vi "Dual_DM_Control_Main_V3.vi"() -> ()   [LabVIEW 2014]
uses:
  Controls/MirrorModes.ctl
  Controls/Standard Action.ctl
  <vilib>/Analysis/baseanly.llb/Mean (DBL).vi
  <vilib>/Utility/file.llb/Write To Spreadsheet File (DBL).vi
  <vilib>/Utility/file.llb/Read From Spreadsheet File (DBL).vi
  <vilib>/Analysis/NI_AALBase.lvlib
panel:
  in  "Active Mirror":enum32{"Mirror 1", "Mirror 2"}(radio)
  in  "Clear Modes":bool
  in  "Mirror Modes":T1
  in  "Load Modes":bool
  in  "Save Modes":bool
  in  "Scan Modes":bool
  in  "Load Flat":bool
  in  "Apply Zero":bool
  in  "Load V Map":bool
  in  "Save V Map":bool
  in  "Apply Flat":bool
  in  "Center Bias":bool
  in  "Exit":bool
  out "Pixel Map (-1 to 1)":dbl[][](graph)
  # "Mode"
  # "Amount (nm)"
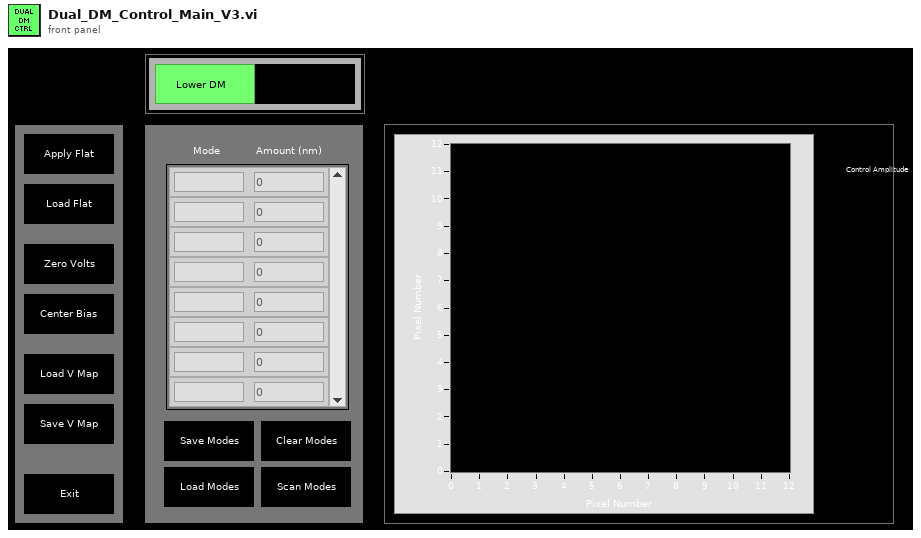
[diagram p1: front panel]
types:
  T1 = typedef "MirrorModes.ctl" = cluster{"Mode":string, "Amplitude":dbl}[]
  T2 = typedef "Standard Action.ctl" = enum16{"Read", "Write"}
  T3 = typedef "MirrorModes_DUAL.ctl" = cluster{"Mode":string, "Amplitude":dbl}[][]
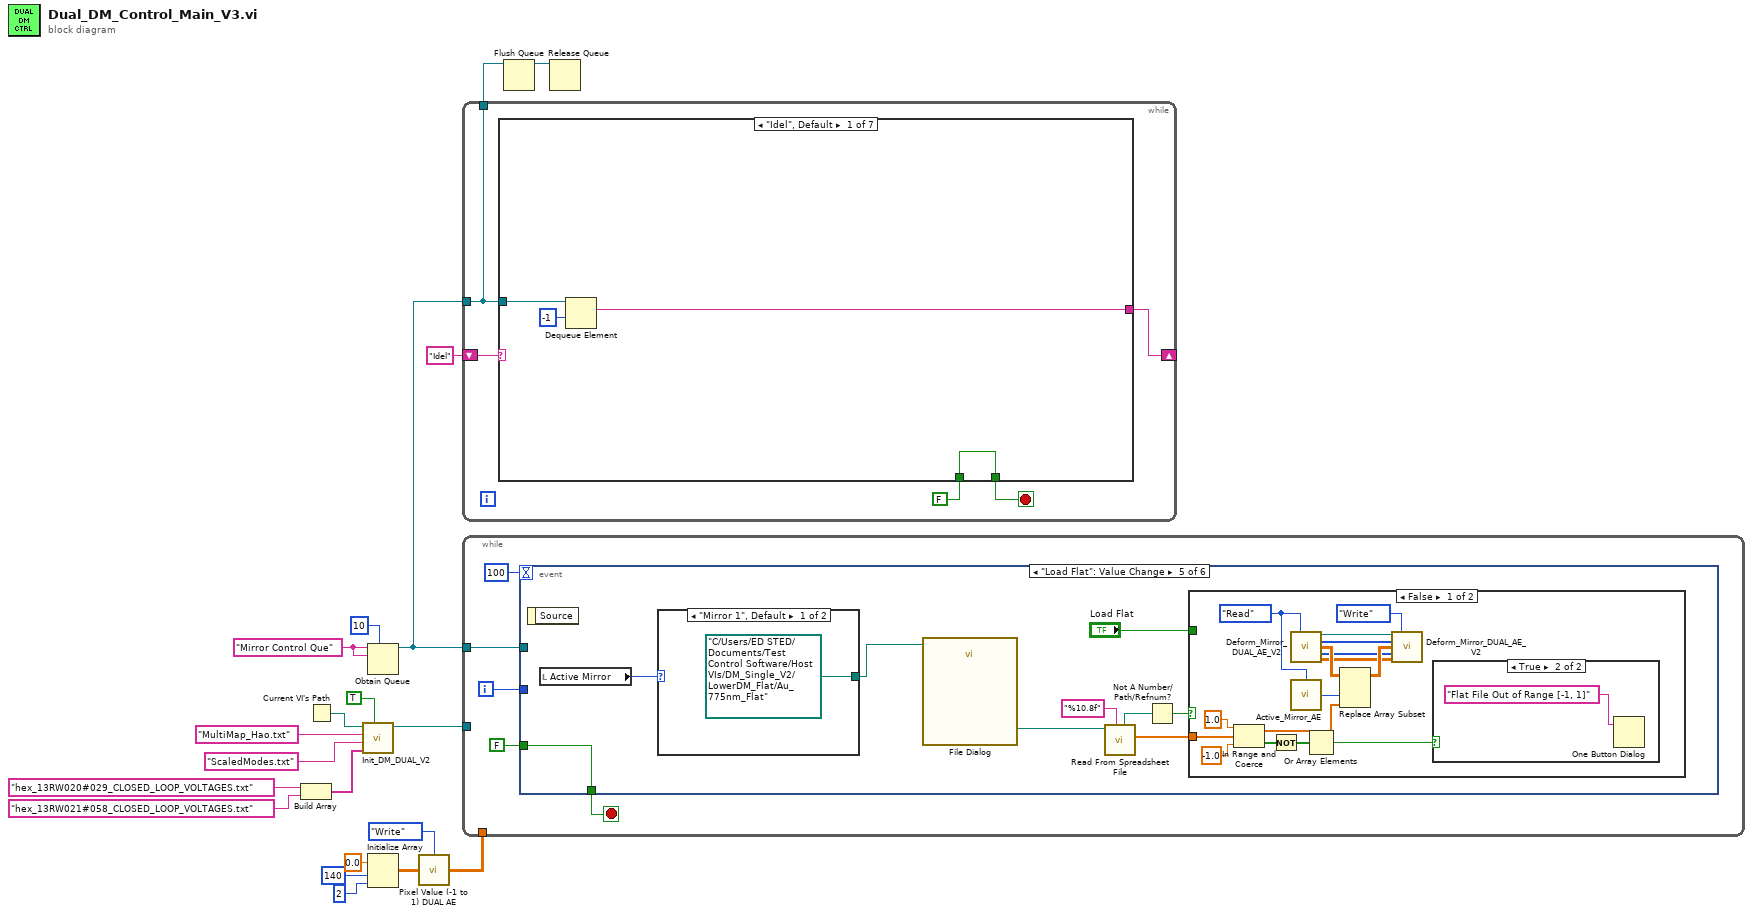
[diagram p0: block diagram]
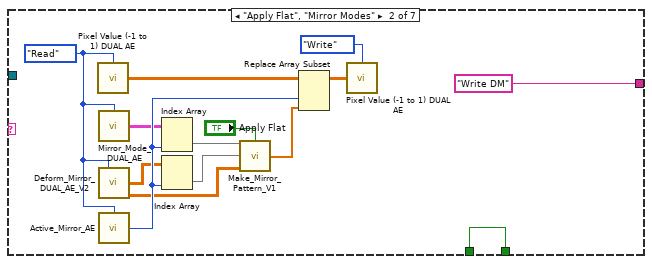
[diagram p2: hidden frame]
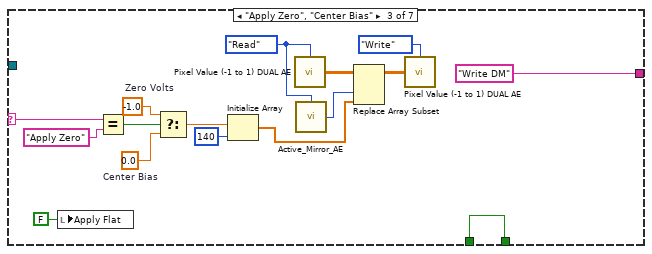
[diagram p3: hidden frame]
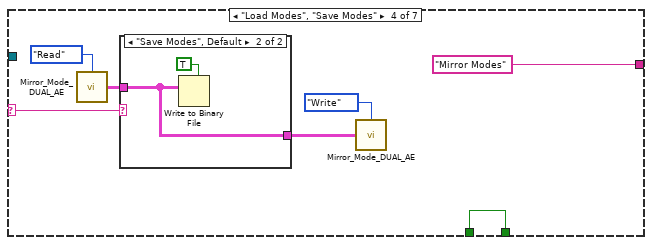
[diagram p4: hidden frame]
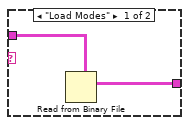
[diagram p5: hidden frame]
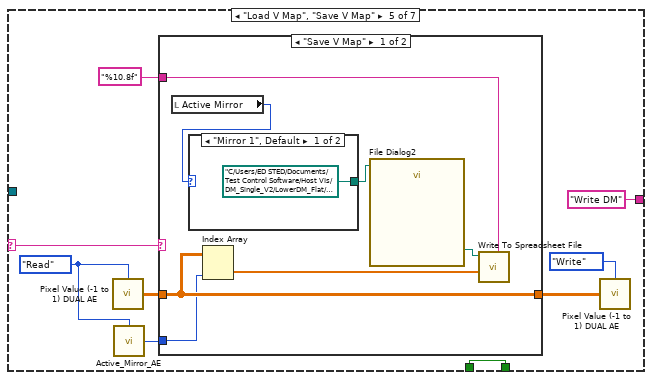
[diagram p6: hidden frame]
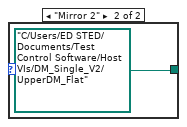
[diagram p7: hidden frame]
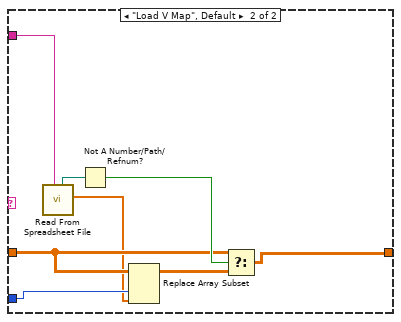
[diagram p8: hidden frame]
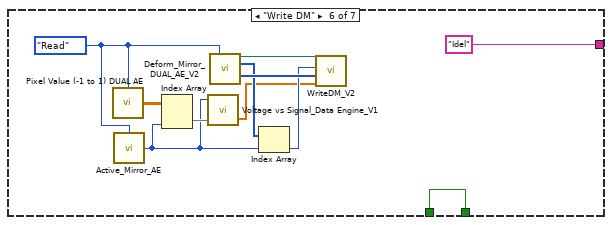
[diagram p9: hidden frame]
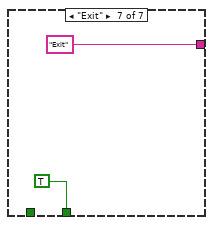
[diagram p10: hidden frame]
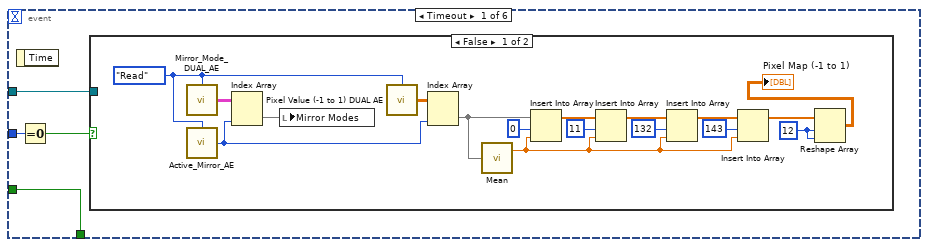
[diagram p11: hidden frame]
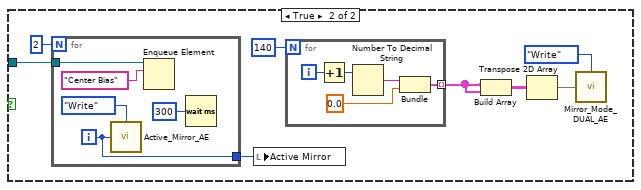
[diagram p12: hidden frame]
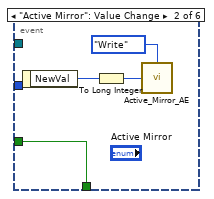
[diagram p13: hidden frame]
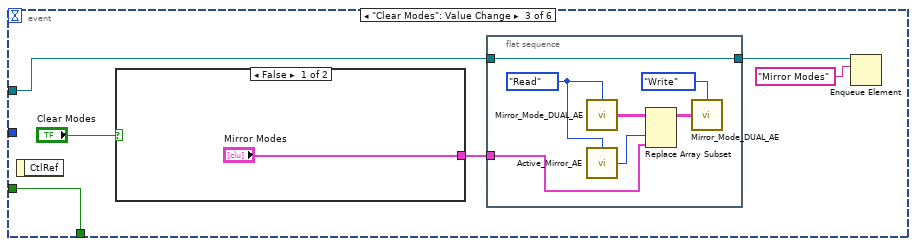
[diagram p14: hidden frame]
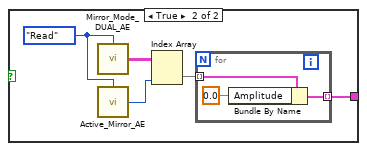
[diagram p15: hidden frame]
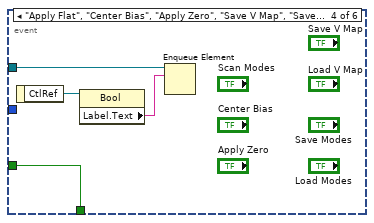
[diagram p16: hidden frame]
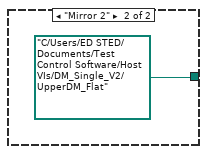
[diagram p17: hidden frame]
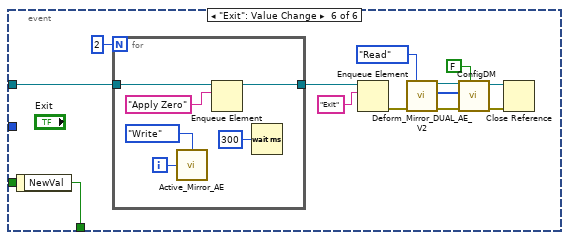
[diagram p20: hidden frame]
diagram:
  w20 = "Mirror Control Que" ("name (unnamed)")
  n1 = Build Array("hex_13RW020#029_CLOSED_LOOP_VOLTAGES.txt" ("name or relative path"), "hex_13RW021#058_CLOSED_LOOP_VOLTAGES.txt" ("name or relative path")) -> (w8:string[])
  n2 = Current VI's Path() -> (path=w12:path)
  n3 = call "Init_DM_DUAL_V2.vi"("BM Flat"=TRUE, "BM Flat File"=w8, "Mirror Modes File"="ScaledModes.txt" ("name or relative path"), "DM Mapping File"="MultiMap_Hao.txt" ("name or relative path"), "Base File Path"=w12) -> ("reference out"=w18:refnum<k7>)  [unwired: 6 in]
  n4 = Obtain Queue(max queue size (-1, unlimited)=10, name (unnamed)=w20, element data type=w20) -> (queue out=w14:refnum<queue>)  [unwired: 2 in, 2 out]
  n5 = Initialize Array(0.0 ("element"), 140 ("dimension size"), 2 ("dimension size")) -> (w4:dbl[][])
  n6 = call "Pixel Value (-1 to 1) DUAL AE.vi"("Action"=Standard_Action."Write", "Pixel Value (-1 to 1)"=w4) -> ("Pixel Value (-1 to 1) Out"=w2:dbl[][])  [unwired: 13 in]
  n7 = while {
    tunnel: w14 -> [w21]
    shift-right: [w25] -> _
    shift-left: "Idel" ("name (unnamed)") -> [w24]
    tunnel: [w21] -> w17
    stop <- w23 stop-if-true
    n8 = case shown="\"Idel\", Default" w24 {
      selector: w24 -> [_ _ w55 w62 w78 _ _]
      tunnel: w21 -> [w29 _ _ _ _ _ _]
      tunnel: [w27 "Write DM" ("name (unnamed)") "Write DM" ("name (unnamed)") "Mirror Modes" ("name (unnamed)") "Write DM" ("name (unnamed)") "Idel" ("name (unnamed)") "Exit" ("name (unnamed)")] -> w25
      tunnel: [w26 w42 w59 w66 w79 w107 TRUE] -> w23
      tunnel: FALSE -> [w26 w42 w59 w66 w79 w107 _]
      frame "Idel", Default {
        n9 = Dequeue Element(queue=w29, timeout in ms (-1)=-1) -> (element=w27:string)  [unwired: 1 in, 3 out]
      }
      frame "Apply Flat", "Mirror Modes" {
        w37 = Standard_Action."Read" ("Action")
        n10 = call "Pixel Value (-1 to 1) DUAL AE.vi"("Action"=w37) -> ("Pixel Value (-1 to 1) Out"=w38:dbl[][])  [unwired: 14 in]
        n11 = call "Mirror_Mode_DUAL_AE.vi"("Action"=w37) -> ("Mirror Modes Out"=w34:T3)  [unwired: 14 in]
        n12 = call "Deform_Mirror_DUAL_AE_V2.vi"("Action"=w37) -> ("Flat Files Out"=w32:dbl[][], "Mode Matrix Out"=w31:dbl[][])  [unwired: 10 in, 3 out]
        n13 = call "Active_Mirror_AE.vi"("Action"=w37) -> ("Active Mirror"=w40:i32)  [unwired: 14 in]
        n14 = Index Array(array=w34, index (col)=w40) -> (element=w35:cluster{"Mode":string, "Amplitude":dbl}[])  [unwired: 1 in]
        n15 = Index Array(array=w32, index (col)=w40) -> (element=w33:dbl[])  [unwired: 1 in]
        n16 = call "Make_Mirror_Pattern_V1.vi"("Mirror Modes In"=w35, "Flat On?"="Apply Flat", "Flat File In"=w33, "Mirror Modes Array"=w31) -> ("Pixel Value U (-1 to 1)"=w39:dbl[])  [unwired: 11 in]
        n17 = Replace Array Subset(array=w38, new element=w39, index (col)=w40) -> (w41:dbl[][])  [unwired: 1 in]
        n18 = call "Pixel Value (-1 to 1) DUAL AE.vi"("Action"=Standard_Action."Write", "Pixel Value (-1 to 1)"=w41) -> ()  [unwired: 13 in, 1 out]
      }
      frame "Apply Zero", "Center Bias" {
        w47 = Standard_Action."Read" ("Action")
        w51 = -1.0  # Zero Volts
        w53 = 0.0  # Center Bias
        n19 = local write "Apply Flat"(FALSE ("Apply Flat")) -> ()
        n20 = Equal?(x=w55, y="Apply Zero") -> (x = y?=w54:bool)
        n21 = Select(t=w51, s=w54, f=w53) -> (s? t:f=w52:dbl)
        n22 = Initialize Array(w52, 140 ("dimension size")) -> (w44:dbl[])
        n23 = call "Pixel Value (-1 to 1) DUAL AE.vi"("Action"=w47) -> ("Pixel Value (-1 to 1) Out"=w45:dbl[][])  [unwired: 14 in]
        n24 = call "Active_Mirror_AE.vi"("Action"=w47) -> ("Active Mirror"=w46:i32)  [unwired: 14 in]
        n25 = Replace Array Subset(array=w45, new element=w44, index (col)=w46) -> (w49:dbl[][])  [unwired: 1 in]
        n26 = call "Pixel Value (-1 to 1) DUAL AE.vi"("Action"=Standard_Action."Write", "Pixel Value (-1 to 1)"=w49) -> ()  [unwired: 13 in, 1 out]
      }
      frame "Load Modes", "Save Modes" {
        n27 = call "Mirror_Mode_DUAL_AE.vi"("Action"=Standard_Action."Read") -> ("Mirror Modes Out"=w61:T3)  [unwired: 14 in]
        n28 = case shown="\"Save Modes\", Default" w62 {
          tunnel: w61 -> [w68 w69]
          tunnel: [w67 w69] -> w60
          frame "Load Modes" {
            n29 = Read from Binary File(5:w68) -> (2:w67:T3)  [unwired: 5 in, 3 out]
          }
          frame "Save Modes", Default {
            n30 = Write to Binary File(data=w69, 5:TRUE ("prepend array or string size? (T)")) -> ()  [unwired: 4 in, 3 out]
          }
        }
        n31 = call "Mirror_Mode_DUAL_AE.vi"("Action"=Standard_Action."Write", "Mirror Modes In"=w60) -> ()  [unwired: 13 in, 1 out]
      }
      frame "Load V Map", "Save V Map" {
        w72 = Standard_Action."Read" ("Action")
        n32 = call "Pixel Value (-1 to 1) DUAL AE.vi"("Action"=w72) -> ("Pixel Value (-1 to 1) Out"=w76:dbl[][])  [unwired: 14 in]
        n33 = call "Active_Mirror_AE.vi"("Action"=w72) -> ("Active Mirror"=w71:i32)  [unwired: 14 in]
        n34 = case shown="\"Save V Map\"" w78 {
          tunnel: w76 -> [w85 w92]
          tunnel: "%10.8f" -> [w86 w96]
          tunnel: [w85 w93] -> w73
          tunnel: w71 -> [w83 w91]
          frame "Save V Map" {
            n35 = local read "Active Mirror"() -> (w81:enum32{"Mirror 1", "Mirror 2"})
            n36 = case shown="\"Mirror 1\", Default" w81 {
              tunnel: [path "C:/Users/ED STED/Documents/Test Control Software/Host VIs/DM_Single_V2/LowerDM_Flat/Au_775nm_Flat" path "C:/Users/ED STED/Documents/Test Control Software/Host VIs/DM_Single_V2/UpperDM_Flat"] -> w80
              frame "Mirror 1", Default {
              }
              frame "Mirror 2" {
              }
            }
            n37 = Index Array(array=w85, index (col)=w83) -> (element=w84:dbl[])  [unwired: 1 in]
            n38 = call "File Dialog2"("start path"=w80) -> ("selected path"=w82:path)  [unwired: 11 in, 3 out]
            n39 = call-poly <vilib>:"Write To Spreadsheet File.vi"("format (%.3f)"=w86, "1D data"=w84, "file path (dialog if empty)"=w82) -> ()  [unwired: 5 in, 1 out]
          }
          frame "Load V Map", Default {
            n40 = call-poly <vilib>:"Read From Spreadsheet File.vi"("format (%.3f)"=w96) -> ("first row"=w90:dbl[], "new file path (Not A Path if cancelled)"=w95:path)  [unwired: 6 in, 3 out]
            n41 = Not A Number/Path/Refnum?(number/path/refnum=w95) -> (NaN/Path/Refnum?=w94:bool)
            n42 = Replace Array Subset(array=w92, new element=w90, index (col)=w91) -> (w89:dbl[][])  [unwired: 1 in]
            n43 = Select(t=w92, s=w94, f=w89) -> (s? t:f=w93:dbl[][])
          }
        }
        n44 = call "Pixel Value (-1 to 1) DUAL AE.vi"("Action"=Standard_Action."Write", "Pixel Value (-1 to 1)"=w73) -> ()  [unwired: 13 in, 1 out]
      }
      frame "Write DM" {
        w102 = Standard_Action."Read" ("Action")
        n45 = call "Pixel Value (-1 to 1) DUAL AE.vi"("Action"=w102) -> ("Pixel Value (-1 to 1) Out"=w103:dbl[][])  [unwired: 14 in]
        n46 = call "Active_Mirror_AE.vi"("Action"=w102) -> ("Active Mirror"=w97:i32)  [unwired: 14 in]
        n47 = Index Array(array=w103, index (col)=w97) -> (element=w98:dbl[])  [unwired: 1 in]
        n48 = call "Voltage vs Signal_Data Engine_V1.vi"("Control Signal In (-1~1)"=w98, "DM #"=w97) -> ("Voltage Out (0~Max. Vol.)"=w99:dbl[])  [unwired: 1 in, 1 out]
        n49 = call "Deform_Mirror_DUAL_AE_V2.vi"("Action"=w102) -> ("Refnum Out"=w105:refnum<k7>, "IDs Out"=w101:i32[], "Multi Map Data Out"=w104:i32[])  [unwired: 10 in, 2 out]
        n50 = Index Array(array=w101, index=w97) -> (element=w100:i32)
        n51 = call "WriteDM_V2.vi"("reference in"=w105, "nDevId"=w100, "MultiDM  Mapping"=w104, "Voltage Array in"=w99) -> ()  [unwired: 2 in, 2 out]
      }
      frame "Exit" {
      }
    }
  }
  n52 = while {
    tunnel: w14 -> [w110]
    tunnel: w18 -> [_]
    tunnel: w2 -> [_]
    i -> [w111]
    stop <- w114 stop-if-true
    n53 = event shown="[4] \"Load Flat\": Value Change" {
      selector: _ -> [_ _ _ _ _ _]
      dyn-events: _ -> [_ _ _ _ _ _]
      timeout: 100 -> [_ _ _ _ _ _]
      tunnel: [w118 w157 w163 w183 w192 w223] -> w114
      tunnel: FALSE -> [w118 w157 w163 w183 w192 _]
      tunnel: w111 -> [w117 _ _ _ _ _]
      tunnel: w110 -> [w115 _ w162 w182 _ w221]
      event Timeout {
        n54 = event-data() -> ()  [unwired: 1 in, 1 out]
        n55 = Equal To 0?(x=w117) -> (x = 0?=w116:bool)
        n56 = case shown="False" w116 {
          tunnel: w115 -> [_ w143]
          frame False {
            w131 = 12 ("dimension size")
            w132 = Standard_Action."Read" ("Action")
            n57 = call "Mirror_Mode_DUAL_AE.vi"("Action"=w132) -> ("Mirror Modes Out"=w119:T3)  [unwired: 14 in]
            n58 = call "Active_Mirror_AE.vi"("Action"=w132) -> ("Active Mirror"=w134:i32)  [unwired: 14 in]
            n59 = Index Array(array=w119, index (col)=w134) -> (element=w120:cluster{"Mode":string, "Amplitude":dbl}[])  [unwired: 1 in]
            n60 = local write "Mirror Modes"(w120) -> ()
            n61 = call "Pixel Value (-1 to 1) DUAL AE.vi"("Action"=w132) -> ("Pixel Value (-1 to 1) Out"=w133:dbl[][])  [unwired: 14 in]
            n62 = Index Array(array=w133, index (col)=w134) -> (element=w135:dbl[])  [unwired: 1 in]
            n63 = call-poly <vilib>:"Mean.vi"("X"=w135) -> ("mean"=w129:dbl)  [unwired: 1 out]
            n64 = Insert Into Array(array=w135, index=0, new element=w129) -> (w124:dbl[])
            n65 = Insert Into Array(array=w124, index=11, new element=w129) -> (w126:dbl[])
            n66 = Insert Into Array(array=w126, index=132, new element=w129) -> (w128:dbl[])
            n67 = Insert Into Array(array=w128, index=143, new element=w129) -> (w121:dbl[])
            n68 = Reshape Array(w121, w131, w131) -> (→"Pixel Map (-1 to 1)":dbl[][])
          }
          frame True {
            n69 = for {
              N: 2 -> [_]
              tunnel: w143 -> [w148]
              tunnel: [w144] -> w136
              i -> [w144]
              n70 = call "Active_Mirror_AE.vi"("Action"=Standard_Action."Write", "Active Mirror In"=w144) -> ()  [unwired: 13 in, 1 out]
              n71 = Enqueue Element(queue=w148, element="Center Bias") -> ()  [unwired: 2 in, 3 out]
              n72 = Wait (ms)(milliseconds to wait=u32 300) -> ()  [unwired: 1 out]
            }
            n73 = local write "Active Mirror"(w136) -> ()
            n74 = for {
              N: 140 -> [_]
              tunnel: [w149] -> w140 mode=indexing
              i -> [w153]
              n75 = Increment(x=w153) -> (x+1=w152:i32)
              n76 = Number To Decimal String(number=w152) -> (decimal integer string=w151:string)  [unwired: 1 in]
              n77 = Bundle(w151, 0.0) -> (w149:cluster{string, dbl})  [unwired: 1 in]
            }
            n78 = Build Array(w140, w140) -> (w138:cluster{string, dbl}[][])
            n79 = Transpose 2D Array(2D array=w138) -> (transposed array=w137:cluster{string, dbl}[][])
            n80 = call "Mirror_Mode_DUAL_AE.vi"("Action"=Standard_Action."Write", "Mirror Modes In"=w137) -> ()  [unwired: 13 in, 1 out]
          }
        }
      }
      event "Active Mirror": Value Change {
        n81 = event-data() -> ("NewVal"=w156:enum32{"Mirror 1", "Mirror 2"})  [unwired: 1 in]
        n82 = To Long Integer(number=w156) -> (32bit integer=w155:i32)
        n83 = call "Active_Mirror_AE.vi"("Action"=Standard_Action."Write", "Active Mirror In"=w155) -> ()  [unwired: 13 in, 1 out]
      }
      event "Clear Modes": Value Change {
        n84 = event-data() -> ()  [unwired: 1 in, 1 out]
        n85 = case shown="False" "Clear Modes" {
          tunnel: ["Mirror Modes" w165] -> w158
          frame False {
          }
          frame True {
            w168 = Standard_Action."Read" ("Action")
            n86 = call "Mirror_Mode_DUAL_AE.vi"("Action"=w168) -> ("Mirror Modes Out"=w167:T3)  [unwired: 14 in]
            n87 = call "Active_Mirror_AE.vi"("Action"=w168) -> ("Active Mirror"=w169:i32)  [unwired: 14 in]
            n88 = Index Array(array=w167, index (col)=w169) -> (element=w166:cluster{"Mode":string, "Amplitude":dbl}[])  [unwired: 1 in]
            n89 = for {
              tunnel: w166 -> [w172] mode=indexing
              tunnel: [w170] -> w165 mode=indexing
              n90 = Bundle By Name(cluster=w172, "Amplitude"=0.0) -> (w170:cluster{"Mode":string, "Amplitude":dbl})
            }
          }
        }
        n91 = flat-sequence {
          tunnel: w158 -> [w173]
          tunnel: w162 -> [w179]
          tunnel: [w179] -> w160
          frame #0 {
            w176 = Standard_Action."Read" ("Action")
            n92 = call "Mirror_Mode_DUAL_AE.vi"("Action"=w176) -> ("Mirror Modes Out"=w175:T3)  [unwired: 14 in]
            n93 = call "Active_Mirror_AE.vi"("Action"=w176) -> ("Active Mirror"=w177:i32)  [unwired: 14 in]
            n94 = Replace Array Subset(array=w175, new element=w173, index (col)=w177) -> (w178:T3)  [unwired: 1 in]
            n95 = call "Mirror_Mode_DUAL_AE.vi"("Action"=Standard_Action."Write", "Mirror Modes In"=w178) -> ()  [unwired: 13 in, 1 out]
          }
        }
        n96 = Enqueue Element(queue=w160, element="Mirror Modes") -> ()  [unwired: 2 in, 3 out]
      }
      event "Apply Flat", "Center Bias", "Apply Zero", "Save V Map", "Save Modes", "Load Modes", "Load V Map", "Scan Modes": Value Change {
        n97 = event-data() -> ("CtlRef"=w181:refnum<vi>)  [unwired: 1 in]
        n98 = property class="Bool"(reference=w181) -> ("Label.Text"=w180:string)  [unwired: 1 in, 2 out]
        n99 = Enqueue Element(queue=w182, element=w180) -> ()  [unwired: 2 in, 3 out]
      }
      event "Load Flat": Value Change {
        n100 = event-data() -> ()  [unwired: 1 in, 1 out]
        n101 = local read "Active Mirror"() -> (w185:enum32{"Mirror 1", "Mirror 2"})
        n102 = case shown="\"Mirror 1\", Default" w185 {
          tunnel: [path "C:/Users/ED STED/Documents/Test Control Software/Host VIs/DM_Single_V2/LowerDM_Flat/Au_775nm_Flat" path "C:/Users/ED STED/Documents/Test Control Software/Host VIs/DM_Single_V2/UpperDM_Flat"] -> w184
          frame "Mirror 1", Default {
          }
          frame "Mirror 2" {
          }
        }
        n103 = call "File Dialog"("start path"=w184) -> ("selected path"=w186:path)  [unwired: 11 in, 3 out]
        n104 = call-poly <vilib>:"Read From Spreadsheet File.vi"("format (%.3f)"="%10.8f", "file path (dialog if empty)"=w186) -> ("first row"=w188:dbl[], "new file path (Not A Path if cancelled)"=w190:path)  [unwired: 5 in, 3 out]
        n105 = Not A Number/Path/Refnum?(number/path/refnum=w190) -> (NaN/Path/Refnum?=w189:bool)
        n106 = case shown="False" w189 {
          tunnel: w188 -> [w210 _]
          tunnel: "Load Flat" -> [_ _]
          frame False {
            w201 = Standard_Action."Read" ("Action")
            n107 = In Range and Coerce(upper limit=1.0, x=w210, lower limit=-1.0) -> (coerced(x)=w195:dbl[], In Range?=w207:bool[])
            n108 = Not(x=w207) -> (.not. x?=w206:bool[])
            n109 = call "Deform_Mirror_DUAL_AE_V2.vi"("Action"=w201) -> ("Refnum Out"=w196:refnum<k7>, "IDs Out"=w197:i32[], "Flat Files Out"=w202:dbl[][], "Multi Map Data Out"=w198:i32[], "Mode Matrix Out"=w199:dbl[][])  [unwired: 10 in]
            n110 = call "Active_Mirror_AE.vi"("Action"=w201) -> ("Active Mirror"=w204:i32)  [unwired: 14 in]
            n111 = Or Array Elements(Boolean array=w206) -> (logical OR=w205:bool)
            n112 = Replace Array Subset(array=w202, new element=w195, index (col)=w204) -> (w203:dbl[][])  [unwired: 1 in]
            n113 = call "Deform_Mirror_DUAL_AE_V2.vi"("Refnum In"=w196, "Action"=Standard_Action."Write", "IDs In"=w197, "Flat Files In"=w203, "Multi Map Data In"=w198, "Mode Matrix"=w199) -> ()  [unwired: 5 in, 5 out]
            n114 = case shown="True" w205 {
              frame False {
              }
              frame True {
                n115 = One Button Dialog(message="Flat File Out of Range [-1, 1]") -> ()  [unwired: 1 in, 1 out]
              }
            }
          }
          frame True {
          }
        }
      }
      event "Exit": Value Change {
        n116 = event-data() -> ("NewVal"=w223:bool)  [unwired: 1 in]
        n117 = for {
          N: 2 -> [_]
          tunnel: w221 -> [w229]
          tunnel: [w224] -> w212
          i -> [w225]
          n118 = call "Active_Mirror_AE.vi"("Action"=Standard_Action."Write", "Active Mirror In"=w225) -> ()  [unwired: 13 in, 1 out]
          n119 = Enqueue Element(queue=w229, element="Apply Zero") -> (queue out=w224:refnum<queue>)  [unwired: 2 in, 2 out]
          n120 = Wait (ms)(milliseconds to wait=u32 300) -> ()  [unwired: 1 out]
        }
        n121 = Enqueue Element(queue=w212, element="Exit") -> (error out=w216:errorcluster)  [unwired: 2 in, 2 out]
        n122 = call "Deform_Mirror_DUAL_AE_V2.vi"("Action"=Standard_Action."Read") -> ("Refnum Out"=w219:refnum<k7>, "IDs Out"=w214:i32[])  [unwired: 10 in, 3 out]
        n123 = call "ConfigDM.vi"("High Voltage"=FALSE, "error in (no error)"=w216, "Dev IDs"=w214, "Automation Refnum in"=w219) -> ("error out"=w215:errorcluster, "Automation Refnum out"=w218:refnum<k7>)  [unwired: 6 in]
        n124 = Close Reference(reference=w218, error in (no error)=w215) -> ()  [unwired: 1 out]
      }
    }
  }
  n125 = Flush Queue(queue=w17) -> (queue out=w16:refnum<queue>)  [unwired: 1 in, 2 out]
  n126 = Release Queue(queue=w16) -> ()  [unwired: 2 in, 3 out]
